vi "ApplyQueuedMapUpdates.vi"(8 "error in (no error)":errorcluster, 11 "AbstractWorldMap in":refnum<class "NI_Robotics_AbstractWorldMap.lvclass">) -> (0 "error out":errorcluster, 3 "AbstractWorldMap out":refnum<class "NI_Robotics_AbstractWorldMap.lvclass">)   [LabVIEW 2017, in "NI_Robotics_AbstractWorldMap.lvclass"]
uses:
  <vilib>/robotics/Navigation/shared/WorldMap/AbstractWorldMap/NI_Robotics_AbstractWorldMap.lvclass
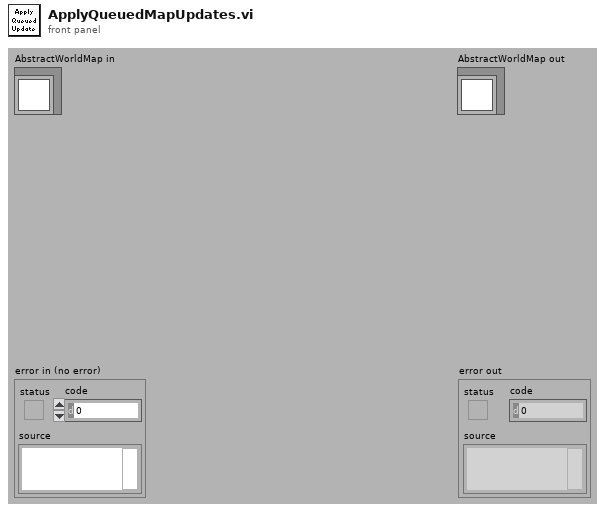
[diagram p1: front panel]
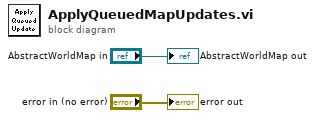
[diagram p0: block diagram]
diagram:
  "error out" <- "error in (no error)"
  "AbstractWorldMap out" <- "AbstractWorldMap in"
